vi "Configure Von Operation.vi"(8 "error in (no error)":errorcluster, 9 "Enable Von Latch (T: Enable)":bool=TRUE, 10 "Von Voltage (0 V)":dbl min=0.0 max=500.0 step=0.01 format="%.2g", 11 "VISA resource name":refnum<visa-resource-name>) -> (0 "error out":errorcluster, 3 "VISA resource name out":refnum<visa-resource-name>)   [LabVIEW 2018, in "BK Precision 8600 Series.lvlib"]
doc: "Configures the Von operation, which control the voltage turn on state for the electronic load. \n\nNote: When the input voltage exceeds the Von voltage value, the electronic load’s input state turns on.\nThis function can protect a DUT when its voltage goes below a specified level."
uses:
  <instrlib>/BK Precision 8600 Series/BK Precision 8600 Series.lvlib
panel:
  # "V"
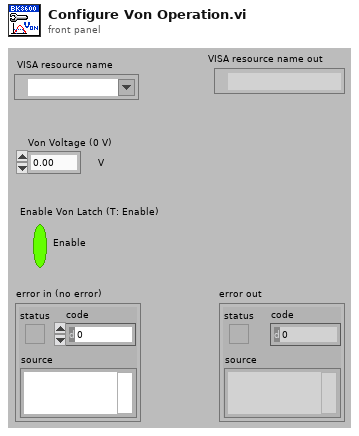
[diagram p1: front panel]
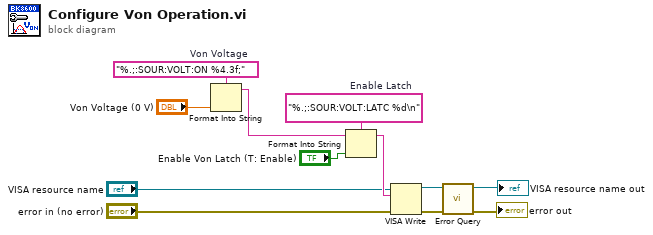
[diagram p0: block diagram]
diagram:
  w6 = "%.;:SOUR:VOLT:ON %4.3f;"  # Von Voltage
  w12 = "%.;:SOUR:VOLT:LATC %d\n"  # Enable Latch
  n1 = Format Into String(format string=w6, "Von Voltage (0 V)") -> (resulting string=w3:string)  [unwired: 2 in, 1 out]
  n2 = Format Into String(format string=w12, initial string=w3, "Enable Von Latch (T: Enable)") -> (resulting string=w9:string)  [unwired: 1 in, 1 out]
  n3 = VISA Write(VISA resource name="VISA resource name", write buffer=w9, error in (no error)="error in (no error)") -> (VISA resource name out=w10:refnum<visa-resource-name>, error out=w11:errorcluster)  [unwired: 1 out]
  n4 = call <instrlib>:"Error Query.vi"("error in (no error)"=w11, "VISA resource name"=w10) -> ("error out"=→"error out":errorcluster, "VISA resource name out"=→"VISA resource name out":refnum<visa-resource-name>)  [unwired: 6 in, 2 out]
